vi "PiezoSetOutputValueTrigger.vi"(8 "error in (no error)":errorcluster, 9 "Período":sgl, 10 "MG17Piezo":refnum<k7>, 11 "amplitude":sgl) -> (0 "error out":errorcluster)   [LabVIEW 2014]
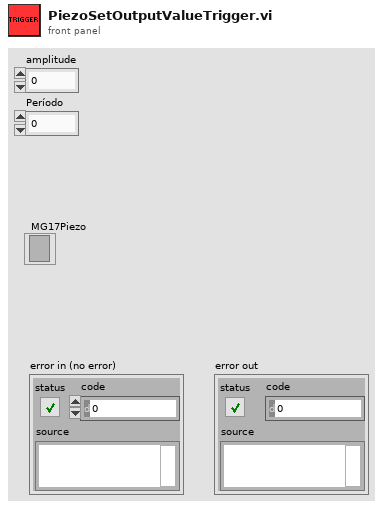
[diagram p1: front panel]
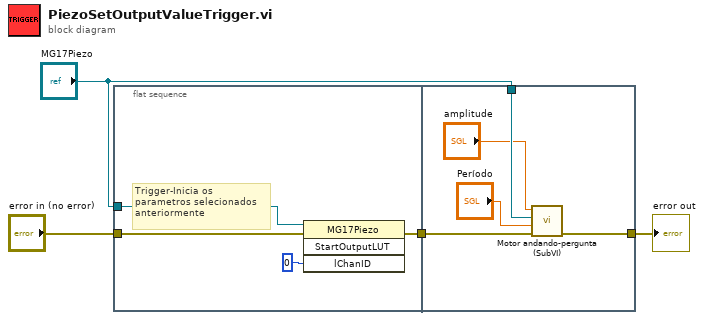
[diagram p0: block diagram]
diagram:
  n1 = flat-sequence {
    tunnel: [w7] -> w4
    tunnel: "MG17Piezo" -> [w6]
    tunnel: "error in (no error)" -> [w5]
    tunnel: w4 -> [w13]
    tunnel: "MG17Piezo" -> [w12]
    tunnel: [w11] -> w3
    frame #0 {
      # "Trigger-Inicia os \nparametros selecionados \nanteriormente"
      n2 = invoke class="MG17Piezo" method="StartOutputLUT"(reference=w6, error in=w5, "lChanID"=0) -> (error out=w7:errorcluster)  [unwired: 1 in, 3 out]
    }
    frame #1 {
      n3 = call "Motor andando-pergunta (SubVI).vi"("error in (no error)"=w13, "Período"="Período", "MG17Piezo"=w12, "amplitude"="amplitude") -> ("error out"=w11:errorcluster)  [unwired: 7 in]
    }
  }
  "error out" <- w3
